vi "我的期末 鋼琴.vi"() -> ()   [LabVIEW 2014]
panel:
  in  "?":bool
  out "Ring 2":i32(ring)
  in  "stop":bool
  in  "高5.5":bool
  in  "高4.5":bool
  in  "高6.5":bool
  in  "高7":bool
  in  "高6":bool
  in  "高5":bool
  in  "高4":bool
  in  "高2.5":bool
  in  "高1.5":bool
  in  "高3":bool
  in  "高2":bool
  in  "高1":bool
  in  "中5.5":bool
  in  "中4.5":bool
  in  "中6.5":bool
  in  "中7":bool
  in  "中6":bool
  in  "中5":bool
  in  "中4":bool
  in  "中音2.5":bool
  in  "中音1.5":bool
  in  "中3":bool
  in  "中音2":bool
  in  "中音1":bool
  in  "低5.5":bool
  in  "低音2.5":bool
  in  "低音4.5":bool
  in  "低音6.5":bool
  in  "低音1.5":bool
  in  "低音7":bool
  in  "低音6":bool
  in  "低音5":bool
  in  "低音4":bool
  in  "低音3":bool
  in  "低音2":bool
  in  "低音1":bool
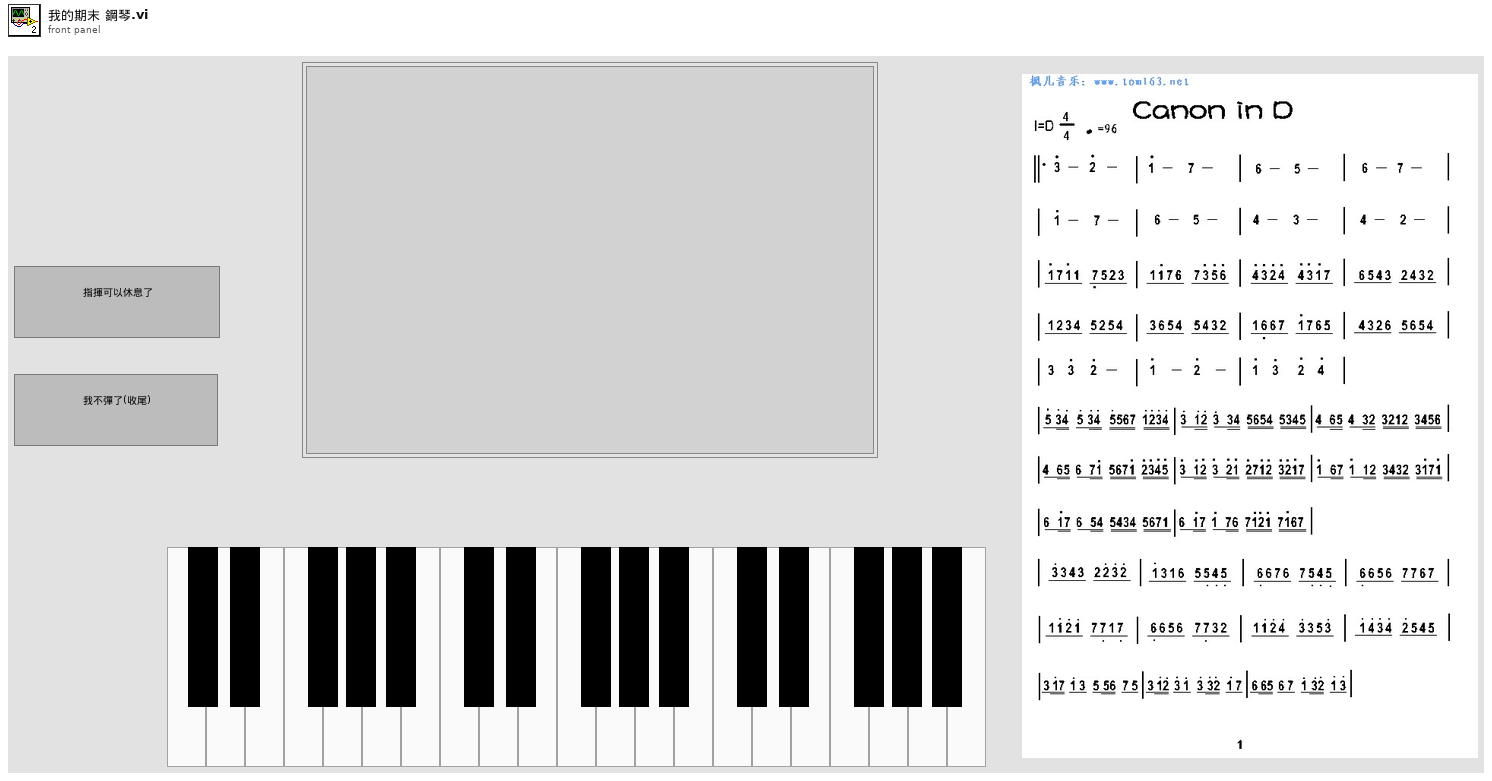
[diagram p1: front panel]
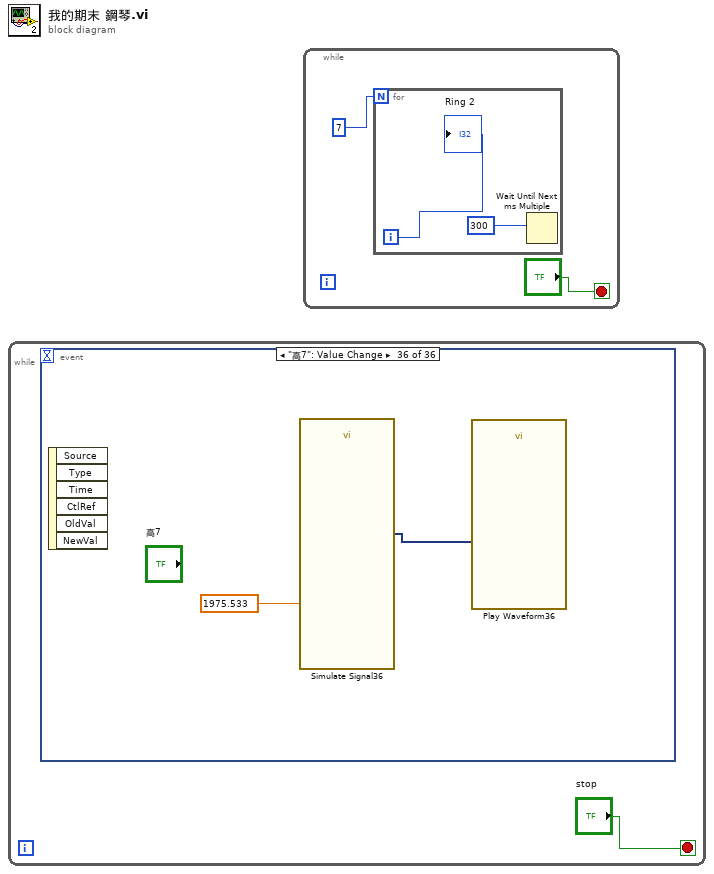
[diagram p0: block diagram]
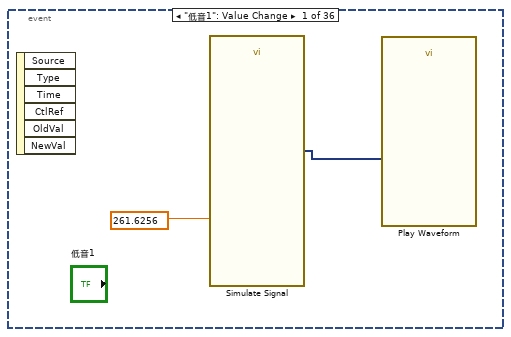
[diagram p2: hidden frame]
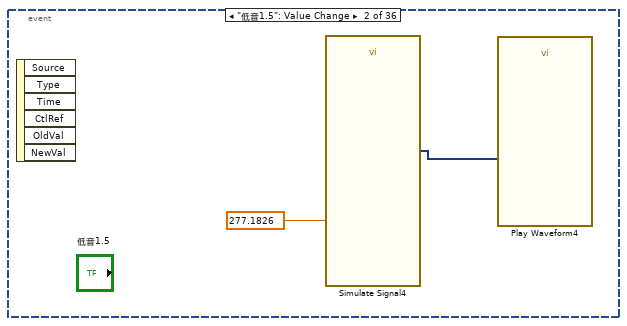
[diagram p3: hidden frame]
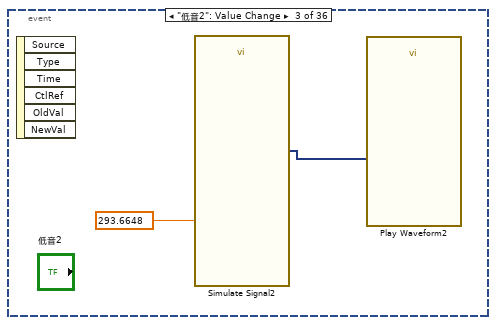
[diagram p4: hidden frame]
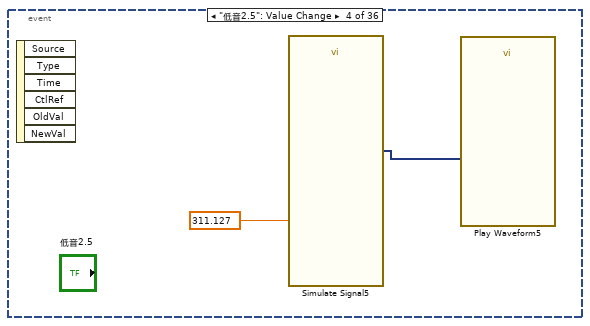
[diagram p5: hidden frame]
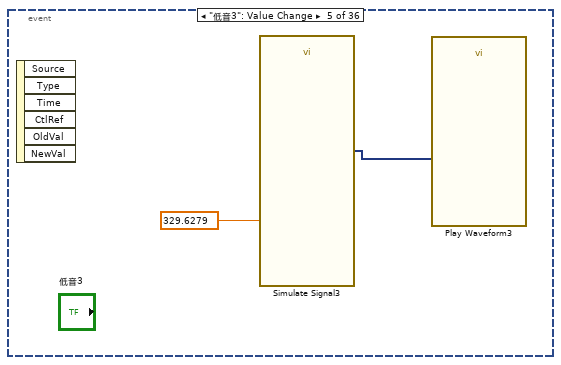
[diagram p6: hidden frame]
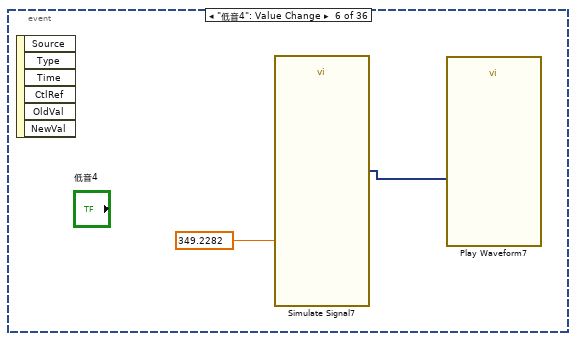
[diagram p7: hidden frame]
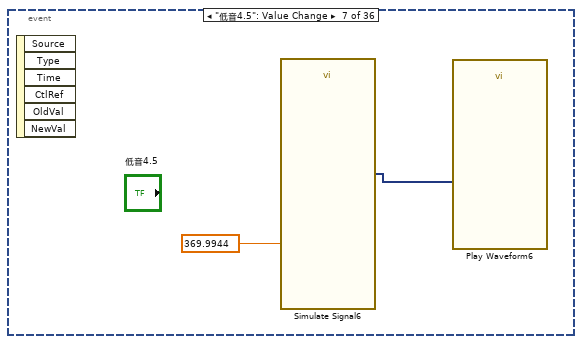
[diagram p8: hidden frame]
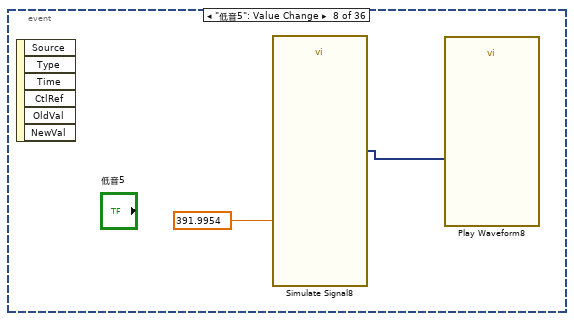
[diagram p9: hidden frame]
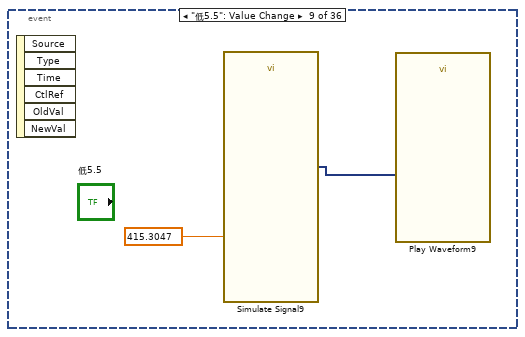
[diagram p10: hidden frame]
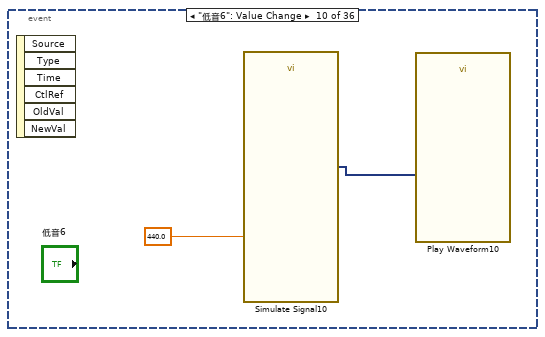
[diagram p11: hidden frame]
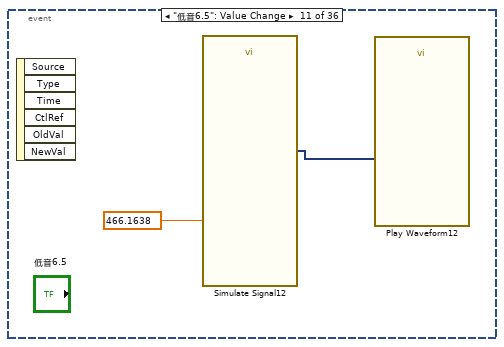
[diagram p12: hidden frame]
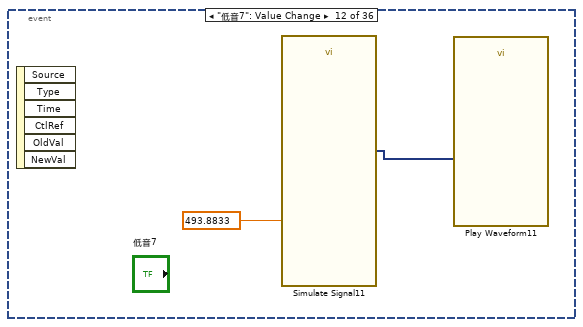
[diagram p13: hidden frame]
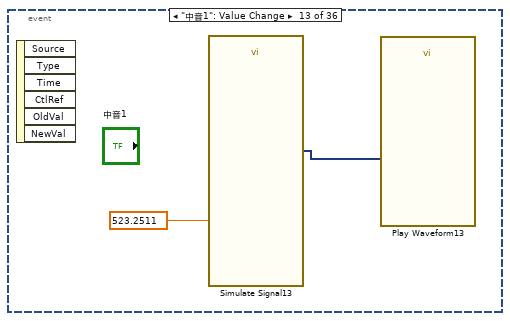
[diagram p14: hidden frame]
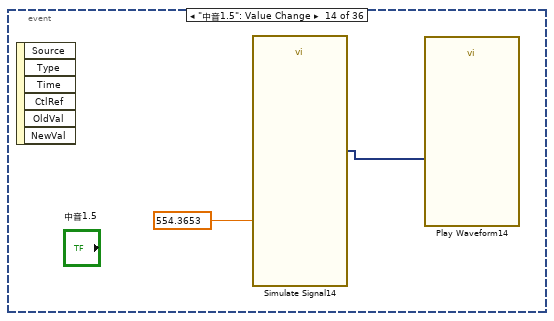
[diagram p15: hidden frame]
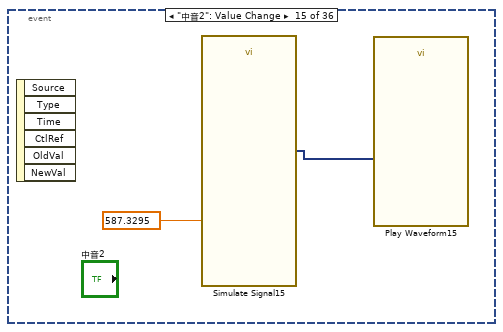
[diagram p16: hidden frame]
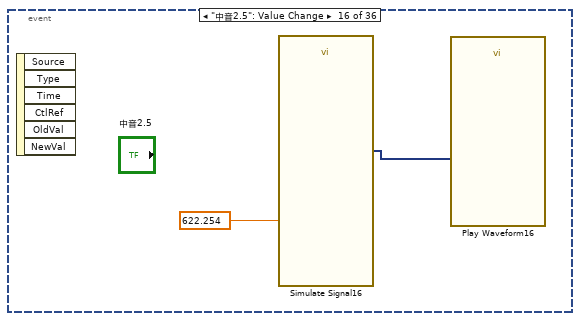
[diagram p17: hidden frame]
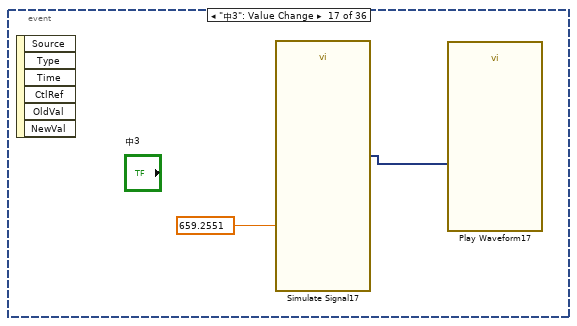
[diagram p18: hidden frame]
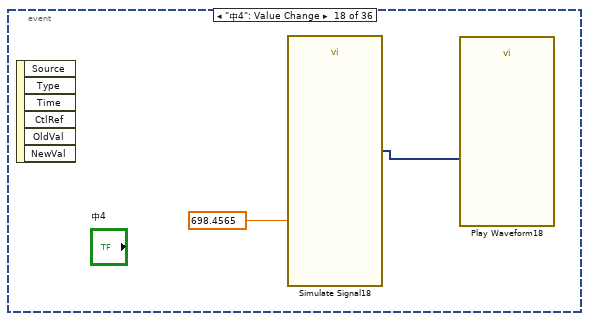
[diagram p19: hidden frame]
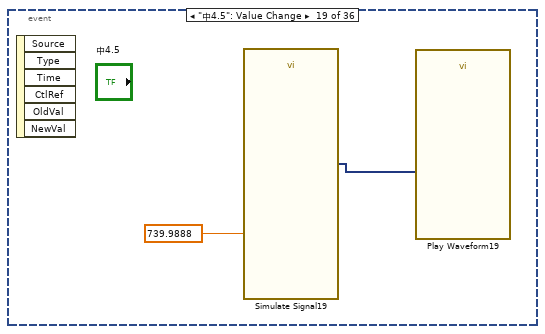
[diagram p20: hidden frame]
diagram:
  n1 = while {
    stop <- "stop" stop-if-true
    n2 = event shown="[35] \"高7\": Value Change" {
      selector: _ -> [_ _ _ _ _ _ _ _ _ _ _ _ _ _ _ _ _ _ _ _ _ _ _ _ _ _ _ _ _ _ _ _ _ _ _ _]
      dyn-events: _ -> [_ _ _ _ _ _ _ _ _ _ _ _ _ _ _ _ _ _ _ _ _ _ _ _ _ _ _ _ _ _ _ _ _ _ _ _]
      timeout: _ -> [_ _ _ _ _ _ _ _ _ _ _ _ _ _ _ _ _ _ _ _ _ _ _ _ _ _ _ _ _ _ _ _ _ _ _ _]
      event "低音1": Value Change {
        n3 = event-data() -> ()  [unwired: 1 in, 6 out]
        n4 = call "Simulate Signal"("Frequency"=261.6256) -> ("Sine"=w2:dynamicdata)  [unwired: 13 in, 1 out]
        n5 = call "Play Waveform"("Data"=w2) -> ()  [unwired: 18 in, 1 out]
      }
      event "低音1.5": Value Change {
        n6 = event-data() -> ()  [unwired: 1 in, 6 out]
        n7 = call "Simulate Signal4"("Frequency"=277.1826) -> ("Sine"=w5:dynamicdata)  [unwired: 13 in, 1 out]
        n8 = call "Play Waveform4"("Data"=w5) -> ()  [unwired: 18 in, 1 out]
      }
      event "低音2": Value Change {
        n9 = event-data() -> ()  [unwired: 1 in, 6 out]
        n10 = call "Simulate Signal2"("Frequency"=293.6648) -> ("Sine"=w7:dynamicdata)  [unwired: 13 in, 1 out]
        n11 = call "Play Waveform2"("Data"=w7) -> ()  [unwired: 18 in, 1 out]
      }
      event "低音2.5": Value Change {
        n12 = event-data() -> ()  [unwired: 1 in, 6 out]
        n13 = call "Simulate Signal5"("Frequency"=311.127) -> ("Sine"=w9:dynamicdata)  [unwired: 13 in, 1 out]
        n14 = call "Play Waveform5"("Data"=w9) -> ()  [unwired: 18 in, 1 out]
      }
      event "低音3": Value Change {
        n15 = event-data() -> ()  [unwired: 1 in, 6 out]
        n16 = call "Simulate Signal3"("Frequency"=329.6279) -> ("Sine"=w11:dynamicdata)  [unwired: 13 in, 1 out]
        n17 = call "Play Waveform3"("Data"=w11) -> ()  [unwired: 18 in, 1 out]
      }
      event "低音4": Value Change {
        n18 = event-data() -> ()  [unwired: 1 in, 6 out]
        n19 = call "Simulate Signal7"("Frequency"=349.2282) -> ("Sine"=w13:dynamicdata)  [unwired: 13 in, 1 out]
        n20 = call "Play Waveform7"("Data"=w13) -> ()  [unwired: 18 in, 1 out]
      }
      event "低音4.5": Value Change {
        n21 = event-data() -> ()  [unwired: 1 in, 6 out]
        n22 = call "Simulate Signal6"("Frequency"=369.9944) -> ("Sine"=w15:dynamicdata)  [unwired: 13 in, 1 out]
        n23 = call "Play Waveform6"("Data"=w15) -> ()  [unwired: 18 in, 1 out]
      }
      event "低音5": Value Change {
        n24 = event-data() -> ()  [unwired: 1 in, 6 out]
        n25 = call "Simulate Signal8"("Frequency"=391.9954) -> ("Sine"=w17:dynamicdata)  [unwired: 13 in, 1 out]
        n26 = call "Play Waveform8"("Data"=w17) -> ()  [unwired: 18 in, 1 out]
      }
      event "低5.5": Value Change {
        n27 = event-data() -> ()  [unwired: 1 in, 6 out]
        n28 = call "Simulate Signal9"("Frequency"=415.3047) -> ("Sine"=w19:dynamicdata)  [unwired: 13 in, 1 out]
        n29 = call "Play Waveform9"("Data"=w19) -> ()  [unwired: 18 in, 1 out]
      }
      event "低音6": Value Change {
        n30 = event-data() -> ()  [unwired: 1 in, 6 out]
        n31 = call "Simulate Signal10"("Frequency"=440.0) -> ("Sine"=w21:dynamicdata)  [unwired: 13 in, 1 out]
        n32 = call "Play Waveform10"("Data"=w21) -> ()  [unwired: 18 in, 1 out]
      }
      event "低音6.5": Value Change {
        n33 = event-data() -> ()  [unwired: 1 in, 6 out]
        n34 = call "Simulate Signal12"("Frequency"=466.1638) -> ("Sine"=w23:dynamicdata)  [unwired: 13 in, 1 out]
        n35 = call "Play Waveform12"("Data"=w23) -> ()  [unwired: 18 in, 1 out]
      }
      event "低音7": Value Change {
        n36 = event-data() -> ()  [unwired: 1 in, 6 out]
        n37 = call "Simulate Signal11"("Frequency"=493.8833) -> ("Sine"=w25:dynamicdata)  [unwired: 13 in, 1 out]
        n38 = call "Play Waveform11"("Data"=w25) -> ()  [unwired: 18 in, 1 out]
      }
      event "中音1": Value Change {
        n39 = event-data() -> ()  [unwired: 1 in, 6 out]
        n40 = call "Simulate Signal13"("Frequency"=523.2511) -> ("Sine"=w27:dynamicdata)  [unwired: 13 in, 1 out]
        n41 = call "Play Waveform13"("Data"=w27) -> ()  [unwired: 18 in, 1 out]
      }
      event "中音1.5": Value Change {
        n42 = event-data() -> ()  [unwired: 1 in, 6 out]
        n43 = call "Simulate Signal14"("Frequency"=554.3653) -> ("Sine"=w28:dynamicdata)  [unwired: 13 in, 1 out]
        n44 = call "Play Waveform14"("Data"=w28) -> ()  [unwired: 18 in, 1 out]
      }
      event "中音2": Value Change {
        n45 = event-data() -> ()  [unwired: 1 in, 6 out]
        n46 = call "Simulate Signal15"("Frequency"=587.3295) -> ("Sine"=w30:dynamicdata)  [unwired: 13 in, 1 out]
        n47 = call "Play Waveform15"("Data"=w30) -> ()  [unwired: 18 in, 1 out]
      }
      event "中音2.5": Value Change {
        n48 = event-data() -> ()  [unwired: 1 in, 6 out]
        n49 = call "Simulate Signal16"("Frequency"=622.254) -> ("Sine"=w32:dynamicdata)  [unwired: 13 in, 1 out]
        n50 = call "Play Waveform16"("Data"=w32) -> ()  [unwired: 18 in, 1 out]
      }
      event "中3": Value Change {
        n51 = event-data() -> ()  [unwired: 1 in, 6 out]
        n52 = call "Simulate Signal17"("Frequency"=659.2551) -> ("Sine"=w34:dynamicdata)  [unwired: 13 in, 1 out]
        n53 = call "Play Waveform17"("Data"=w34) -> ()  [unwired: 18 in, 1 out]
      }
      event "中4": Value Change {
        n54 = event-data() -> ()  [unwired: 1 in, 6 out]
        n55 = call "Simulate Signal18"("Frequency"=698.4565) -> ("Sine"=w36:dynamicdata)  [unwired: 13 in, 1 out]
        n56 = call "Play Waveform18"("Data"=w36) -> ()  [unwired: 18 in, 1 out]
      }
      event "中4.5": Value Change {
        n57 = event-data() -> ()  [unwired: 1 in, 6 out]
        n58 = call "Simulate Signal19"("Frequency"=739.9888) -> ("Sine"=w38:dynamicdata)  [unwired: 13 in, 1 out]
        n59 = call "Play Waveform19"("Data"=w38) -> ()  [unwired: 18 in, 1 out]
      }
      event "中5": Value Change {
        n60 = event-data() -> ()  [unwired: 1 in, 6 out]
        n61 = call "Simulate Signal20"("Frequency"=783.9909) -> ("Sine"=w40:dynamicdata)  [unwired: 13 in, 1 out]
        n62 = call "Play Waveform20"("Data"=w40) -> ()  [unwired: 18 in, 1 out]
      }
      event "中5.5": Value Change {
        n63 = event-data() -> ()  [unwired: 1 in, 6 out]
        n64 = call "Simulate Signal21"("Frequency"=830.6094) -> ("Sine"=w42:dynamicdata)  [unwired: 13 in, 1 out]
        n65 = call "Play Waveform21"("Data"=w42) -> ()  [unwired: 18 in, 1 out]
      }
      event "中6": Value Change {
        n66 = event-data() -> ()  [unwired: 1 in, 6 out]
        n67 = call "Simulate Signal22"("Frequency"=880.0) -> ("Sine"=w44:dynamicdata)  [unwired: 13 in, 1 out]
        n68 = call "Play Waveform22"("Data"=w44) -> ()  [unwired: 18 in, 1 out]
      }
      event "中6.5": Value Change {
        n69 = event-data() -> ()  [unwired: 1 in, 6 out]
        n70 = call "Simulate Signal23"("Frequency"=932.3275) -> ("Sine"=w46:dynamicdata)  [unwired: 13 in, 1 out]
        n71 = call "Play Waveform23"("Data"=w46) -> ()  [unwired: 18 in, 1 out]
      }
      event "中7": Value Change {
        n72 = event-data() -> ()  [unwired: 1 in, 6 out]
        n73 = call "Simulate Signal24"("Frequency"=987.7666) -> ("Sine"=w48:dynamicdata)  [unwired: 13 in, 1 out]
        n74 = call "Play Waveform24"("Data"=w48) -> ()  [unwired: 18 in, 1 out]
      }
      event "高1": Value Change {
        n75 = event-data() -> ()  [unwired: 1 in, 6 out]
        n76 = call "Simulate Signal25"("Frequency"=1046.505) -> ("Sine"=w50:dynamicdata)  [unwired: 13 in, 1 out]
        n77 = call "Play Waveform25"("Data"=w50) -> ()  [unwired: 18 in, 1 out]
      }
      event "高1.5": Value Change {
        n78 = event-data() -> ()  [unwired: 1 in, 6 out]
        n79 = call "Simulate Signal26"("Frequency"=1108.731) -> ("Sine"=w52:dynamicdata)  [unwired: 13 in, 1 out]
        n80 = call "Play Waveform26"("Data"=w52) -> ()  [unwired: 18 in, 1 out]
      }
      event "高2": Value Change {
        n81 = event-data() -> ()  [unwired: 1 in, 6 out]
        n82 = call "Simulate Signal27"("Frequency"=1174.659) -> ("Sine"=w54:dynamicdata)  [unwired: 13 in, 1 out]
        n83 = call "Play Waveform27"("Data"=w54) -> ()  [unwired: 18 in, 1 out]
      }
      event "高2.5": Value Change {
        n84 = event-data() -> ()  [unwired: 1 in, 6 out]
        n85 = call "Simulate Signal28"("Frequency"=1244.508) -> ("Sine"=w56:dynamicdata)  [unwired: 13 in, 1 out]
        n86 = call "Play Waveform28"("Data"=w56) -> ()  [unwired: 18 in, 1 out]
      }
      event "高3": Value Change {
        n87 = event-data() -> ()  [unwired: 1 in, 6 out]
        n88 = call "Simulate Signal29"("Frequency"=1318.51) -> ("Sine"=w58:dynamicdata)  [unwired: 13 in, 1 out]
        n89 = call "Play Waveform29"("Data"=w58) -> ()  [unwired: 18 in, 1 out]
      }
      event "高4": Value Change {
        n90 = event-data() -> ()  [unwired: 1 in, 6 out]
        n91 = call "Simulate Signal30"("Frequency"=1396.913) -> ("Sine"=w60:dynamicdata)  [unwired: 13 in, 1 out]
        n92 = call "Play Waveform30"("Data"=w60) -> ()  [unwired: 18 in, 1 out]
      }
      event "高4.5": Value Change {
        n93 = event-data() -> ()  [unwired: 1 in, 6 out]
        n94 = call "Simulate Signal31"("Frequency"=1479.978) -> ("Sine"=w62:dynamicdata)  [unwired: 13 in, 1 out]
        n95 = call "Play Waveform31"("Data"=w62) -> ()  [unwired: 18 in, 1 out]
      }
      event "高5": Value Change {
        n96 = event-data() -> ()  [unwired: 1 in, 6 out]
        n97 = call "Simulate Signal32"("Frequency"=1567.982) -> ("Sine"=w64:dynamicdata)  [unwired: 13 in, 1 out]
        n98 = call "Play Waveform32"("Data"=w64) -> ()  [unwired: 18 in, 1 out]
      }
      event "高5.5": Value Change {
        n99 = event-data() -> ()  [unwired: 1 in, 6 out]
        n100 = call "Simulate Signal33"("Frequency"=1661.219) -> ("Sine"=w66:dynamicdata)  [unwired: 13 in, 1 out]
        n101 = call "Play Waveform33"("Data"=w66) -> ()  [unwired: 18 in, 1 out]
      }
      event "高6": Value Change {
        n102 = event-data() -> ()  [unwired: 1 in, 6 out]
        n103 = call "Simulate Signal34"("Frequency"=1760.0) -> ("Sine"=w68:dynamicdata)  [unwired: 13 in, 1 out]
        n104 = call "Play Waveform34"("Data"=w68) -> ()  [unwired: 18 in, 1 out]
      }
      event "高6.5": Value Change {
        n105 = event-data() -> ()  [unwired: 1 in, 6 out]
        n106 = call "Simulate Signal35"("Frequency"=1864.655) -> ("Sine"=w70:dynamicdata)  [unwired: 13 in, 1 out]
        n107 = call "Play Waveform35"("Data"=w70) -> ()  [unwired: 18 in, 1 out]
      }
      event "高7": Value Change {
        n108 = event-data() -> ()  [unwired: 1 in, 6 out]
        n109 = call "Simulate Signal36"("Frequency"=1975.533) -> ("Sine"=w72:dynamicdata)  [unwired: 13 in, 1 out]
        n110 = call "Play Waveform36"("Data"=w72) -> ()  [unwired: 18 in, 1 out]
      }
    }
  }
  n111 = while {
    stop <- "?" stop-if-true
    n112 = for {
      N: 7 -> [_]
      i -> [w76]
      n113 = Wait Until Next ms Multiple(millisecond multiple=300) -> ()  [unwired: 1 out]
      "Ring 2" <- w76
    }
  }
